vi "Oven.vi"() -> ()   [LabVIEW 2021]
panel:
  out "Front L":bool
  out "Rear L":bool
  out "Rear R":bool
  out "Front R":bool
  out "Oven ON Light":bool
  out "Oven Temp":dbl
  in  "Rear R":dbl(knob) scale=0.0..10.0
  in  "Front R":dbl(knob) scale=0.0..10.0
  in  "Oven":dbl(knob) scale=0.0..400.0
  in  "Rear L":dbl(knob) scale=0.0..10.0
  in  "Front L":dbl(knob) scale=0.0..10.0
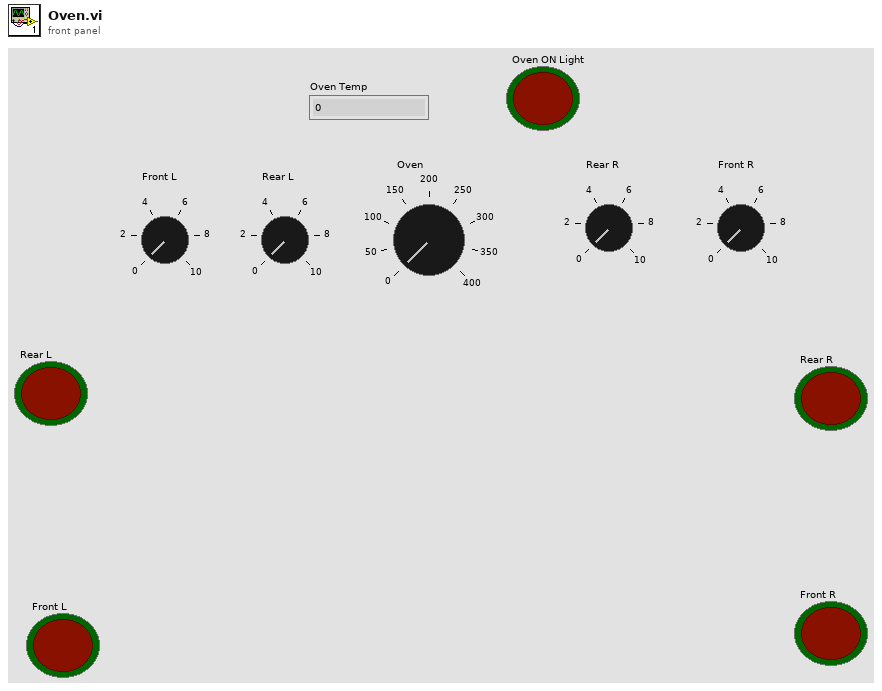
[diagram p1: front panel]
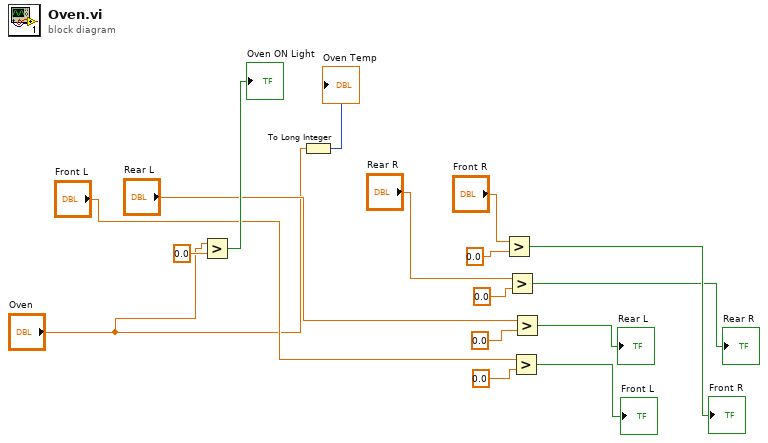
[diagram p0: block diagram]
diagram:
  n1 = Greater?(x="Oven", y=0.0) -> (0:→"Oven ON Light":bool)
  n2 = To Long Integer(number="Oven") -> (32bit integer=→"Oven Temp":i32)
  n3 = Greater?(x="Front R", y=0.0) -> (0:→"Front R":bool)
  n4 = Greater?(x="Rear R", y=0.0) -> (0:→"Rear R":bool)
  n5 = Greater?(x="Front L", y=0.0) -> (0:→"Front L":bool)
  n6 = Greater?(x="Rear L", y=0.0) -> (0:→"Rear L":bool)
